vi "Periodic Tasks.vi"(8 "error in":errorcluster) -> ()   [LabVIEW 2019]
doc: "This VI runs in parallel to other tasks. It can contain as many user-defined periodic loops as you need. These can carry out PID or other sorts of timed response."
uses:
  Robot Global Data.vi
  <vilib>/Rock Robotics/Network Tables/NT Write Number.vi
  <vilib>/Rock Robotics/Network Tables/NT Read Number.vi
  <vilib>/Rock Robotics/Network Tables/NT Write Boolean.vi
  <vilib>/Rock Robotics/WPI/RobotDrive/WPI_RobotDriveArcadeDrive_Standard(NoSaturation).vi
  <vilib>/Rock Robotics/WPI/DriverStation/WPI_DriverStationRobotMode2.ctl
  <vilib>/Rock Robotics/Network Tables/NT Read Boolean.vi
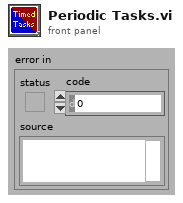
[diagram p1: front panel]
types:
  T1 = typedef "WPI_JoystickDevRef.ctl" = cluster{"Device":T2}
  T2 = typedef "WPI_JoystickDeviceEnum.ctl" = enum16{"USB 0", "USB 1", "USB 2", "USB 3", "USB 4", "USB 5"}
  T3 = typedef "WPI_RobotDriveDevRef.ctl" = cluster{"DevStatus":errorcluster, "Motors[]":T4[], "Square Inputs":bool, "Max Output":dbl}
  T4 = typedef "WPI_MotorControlDeviceRef.ctl" = cluster{"DeviceStatus":errorcluster, "Type":T5, "PWM":cluster{"PWM Channel":T6, "DeadBand":T7}, "CAN":cluster{"Device Number":u8, "SetOutput VI Ref":variant, "GetOutput VI Ref":variant, "Enable VI Ref":variant, "Disable VI Ref":variant, "Data":variant}, "Invert":bool, "DIO PWM":cluster{"PWM \"Enable\" Channel":T6, "DIOChannel":T8, "PWM Rate":dbl}}
  T5 = typedef "WPI_MotorControlType.ctl" = enum16{"PWM", "CAN", "DIO PWM"}
  T6 = typedef "FPGA_DIOPWMChannel.ctl" = enum8{"PWM 0", "PWM 1", "PWM 2", "PWM 3", "PWM 4", "PWM 5", "PWM 6", "PWM 7", "PWM 8", "PWM 9", "PWM MXP 0", "PWM MXP 1", "PWM MXP 2", "PWM MXP 3", "PWM MXP 4", "PWM MXP 5", "PWM MXP 6", "PWM MXP 7", "PWM MXP 8", "PWM MXP 9", "Invalid"}
  T7 = typedef "WPI_PWMDeadband.ctl" = cluster{"Name":string, "maxPositivePwm":i32, "minPositivePwm":i32, "centerPwm":i32, "maxNegativePwm":i32, "minNegativePwm":i32, "angularRange":u16}
  T8 = typedef "FPGA_DIOChannel.ctl" = enum8{"DIO 0", "DIO 1", "DIO 2", "DIO 3", "DIO 4", "DIO 5", "DIO 6", "DIO 7", "DIO 8", "DIO 9", "DIO MXP 0", "DIO MXP 1", "DIO MXP 2", "DIO MXP 3", "DIO MXP 4", "DIO MXP 5", "DIO MXP 6", "DIO MXP 7", "DIO MXP 8", "DIO MXP 9", "DIO MXP 10", "DIO MXP 11", "DIO MXP 12", "DIO MXP 13", "DIO MXP 14", "DIO MXP 15", "SPI Port CS1", "SPI Port CS2", "SPI Port CS3", "SPI Port MISO", "SPI Port MOSI", "Invalid"}
  T9 = cluster{"JoystickDevRef":T1, "RobotDriveDevRef":T3}
  T10 = typedef "WPI_DriverStationRobotMode2.ctl" = enum16{"Autonomous Disabled", "Autonomous Enabled", "Teleop Disabled", "Teleop Enabled", "Disconnected", "Finish", "Test Disabled", "Test Enabled", "Emergency Stopped"}
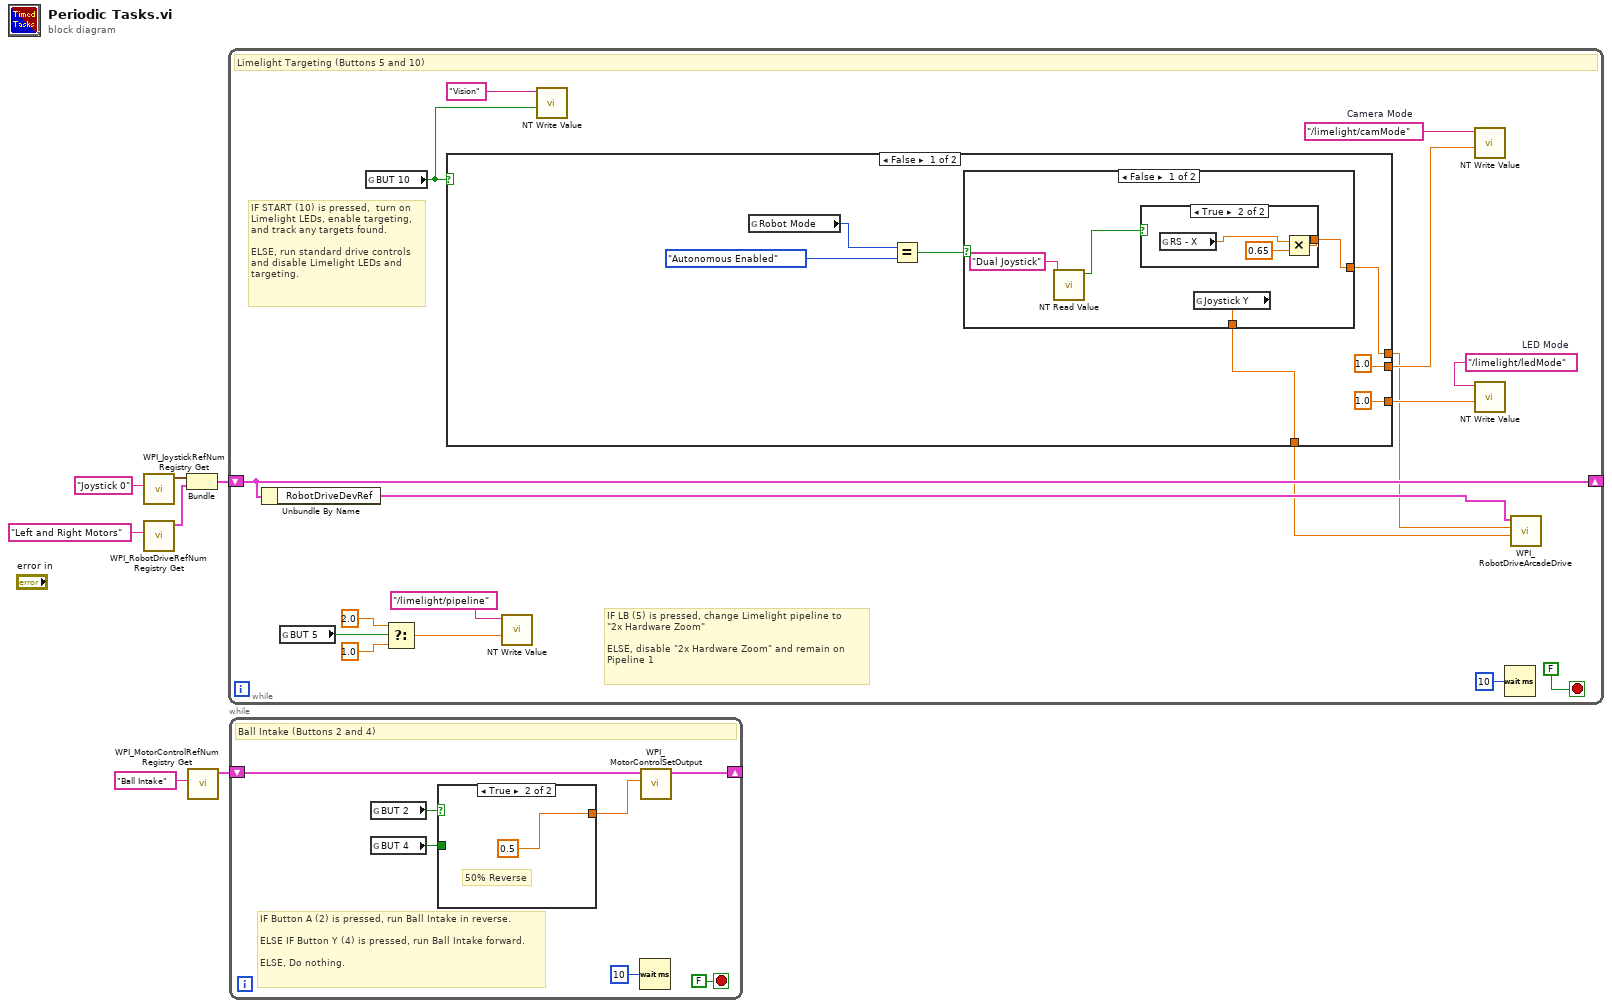
[diagram p0: block diagram]
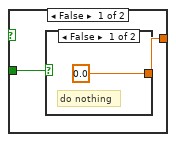
[diagram p2: hidden frame]
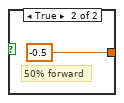
[diagram p3: hidden frame]
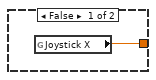
[diagram p4: hidden frame]
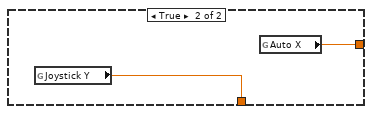
[diagram p5: hidden frame]
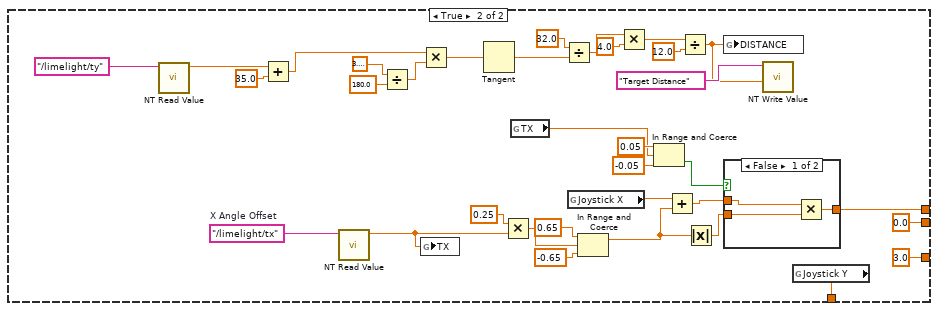
[diagram p6: hidden frame]
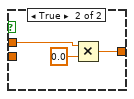
[diagram p7: hidden frame]
diagram:
  n1 = call <vilib>:"WPI_JoystickRefNum Registry Get.vi"("refnum name"="Joystick 0") -> ("JoystickDevRef"=w5:T1)  [unwired: 1 in, 9 out]
  n2 = call <vilib>:"WPI_RobotDriveRefNum Registry Get.vi"("refnum name"="Left and Right Motors") -> ("RobotDriveDevRef"=w4:T3)  [unwired: 1 in, 9 out]
  n3 = Bundle("JoystickDevRef"=w5, "RobotDriveDevRef"=w4) -> (w3:T9)  [unwired: 1 out]
  n4 = call <vilib>:"WPI_MotorControlRefNum Registry Get.vi"("refnum name"="Ball Intake") -> ("MotorControlDevRef"=w2:T4)  [unwired: 9 in, 1 out]
  n5 = while {
    shift-right: [w23] -> _
    shift-left: w3 -> [w23]
    stop <- FALSE stop-if-true
    w20 = "/limelight/camMode"  # Camera Mode
    w21 = "/limelight/ledMode"  # LED Mode
    # "IF LB (5) is pressed, change Limelight pipeline to \n\"2x Hardware Zoom\"\n\nELSE, disable \"2x Hardware Zoom\" and remain on\nPipeline 1"
    # "IF START (10) is pressed,  turn on\nLimelight LEDs, enable targeting,\nand track any targets found.\n\nELSE, run standard drive controls\nand disable Limelight LEDs and \ntargeting."
    # "Limelight Targeting (Buttons 5 and 10)"
    n6 = Unbundle By Name(w23) -> ("RobotDriveDevRef"=w22:T3)
    n7 = global read "Robot Global Data.vi" "BUT 5"() -> (w10:bool)
    n8 = global read "Robot Global Data.vi" "BUT 10"() -> (w16:bool)
    n9 = Select(t=2.0, s=w10, f=1.0) -> (s? t:f=w13:dbl)
    n10 = case shown="False" w16 {
      tunnel: [1.0 ("Numeric") 0.0 ("Numeric")] -> w19
      tunnel: [1.0 ("Numeric") 3.0 ("Numeric")] -> w18
      tunnel: [w25 w52] -> w8
      tunnel: [w29 w51] -> w9
      frame False {
        n11 = global read "Robot Global Data.vi" "Robot Mode"() -> (w28:T10)
        n12 = Equal?(x=w28, y=WPI_DriverStationRobotMode2."Autonomous Enabled") -> (x = y?=w26:bool)
        n13 = case shown="False" w26 {
          tunnel: [w33 w41] -> w29
          tunnel: [w32 w40] -> w25
          frame False {
            n14 = call-poly <vilib>:"NT Read Value.vi"("Name"="Dual Joystick") -> ("Boolean"=w34:bool)  [unwired: 9 in, 1 out]
            n15 = case shown="True" w34 {
              tunnel: [w36 w37] -> w32
              frame False {
                n16 = global read "Robot Global Data.vi" "Joystick X"() -> (w36:dbl)
              }
              frame True {
                n17 = global read "Robot Global Data.vi" "RS - X"() -> (w38:dbl)
                n18 = Multiply(x=w38, y=0.65) -> (x*y=w37:dbl)
              }
            }
            n19 = global read "Robot Global Data.vi" "Joystick Y"() -> (w33:dbl)
          }
          frame True {
            n20 = global read "Robot Global Data.vi" "Joystick Y"() -> (w41:dbl)
            n21 = global read "Robot Global Data.vi" "Auto X"() -> (w40:dbl)
          }
        }
      }
      frame True {
        w53 = "/limelight/tx"  # X Angle Offset
        n22 = call-poly <vilib>:"NT Read Value.vi"("Name"="/limelight/ty") -> ("Numeric"=w68:dbl)  [unwired: 9 in, 1 out]
        n23 = Add(x=w68, y=35.0) -> (x+y=w66:dbl)
        n24 = call-poly <vilib>:"NT Read Value.vi"("Name"=w53) -> ("Numeric"=w57:dbl)  [unwired: 9 in, 1 out]
        n25 = Divide(x=3.141592653589793, y=180.0) -> (x/y=w69:dbl)
        n26 = Multiply(x=w66, y=w69) -> (x*y=w65:dbl)
        n27 = global write "Robot Global Data.vi" "TX"(w57) -> ()
        n28 = Tangent(1:w65) -> (0:w75:dbl)
        n29 = Multiply(x=0.25 ("y"), y=w57) -> (x*y=w54:dbl)
        n30 = global read "Robot Global Data.vi" "TX"() -> (w47:dbl)
        n31 = Divide(x=32.0, y=w75) -> (x/y=w64:dbl)
        n32 = global read "Robot Global Data.vi" "Joystick X"() -> (w45:dbl)
        n33 = In Range and Coerce(upper limit=0.65, x=w54, lower limit=-0.65) -> (coerced(x)=w42:dbl)  [unwired: 1 out]
        n34 = Multiply(x=w64, y=4.0) -> (x*y=w62:dbl)
        n35 = In Range and Coerce(upper limit=0.05, x=w47, lower limit=-0.05) -> (In Range?=w50:bool)  [unwired: 1 out]
        n36 = Add(x=w45, y=w42) -> (x+y=w44:dbl)
        n37 = Divide(x=w62, y=12.0) -> (x/y=w58:dbl)
        n38 = Absolute Value(x=w42) -> (abs(x)=w43:dbl)
        n39 = global write "Robot Global Data.vi" "DISTANCE"(w58) -> ()
        n40 = case shown="False" w50 {
          tunnel: [w78 w80] -> w52
          tunnel: w44 -> [w77 w79]
          tunnel: w43 -> [w76 _]
          frame False {
            n41 = Multiply(x=w77, y=w76) -> (x*y=w78:dbl)
          }
          frame True {
            n42 = Multiply(x=w79, y=0.0) -> (x*y=w80:dbl)
          }
        }
        n43 = call-poly <vilib>:"NT Write Value.vi"("Numeric"=w58, "Name"="Target Distance") -> ()  [unwired: 9 in, 1 out]
        n44 = global read "Robot Global Data.vi" "Joystick Y"() -> (w51:dbl)
      }
    }
    n45 = call-poly <vilib>:"NT Write Value.vi"("Numeric"=w13, "Name"="/limelight/pipeline") -> ()  [unwired: 9 in, 1 out]
    n46 = call-poly <vilib>:"NT Write Value.vi"("Boolean"=w16, "Name"="Vision") -> ()  [unwired: 9 in, 1 out]
    n47 = call-poly <vilib>:"NT Write Value.vi"("Numeric"=w19, "Name"=w20) -> ()  [unwired: 9 in, 1 out]
    n48 = call-poly <vilib>:"NT Write Value.vi"("Numeric"=w18, "Name"=w21) -> ()  [unwired: 9 in, 1 out]
    n49 = Wait (ms)(milliseconds to wait=u32 10) -> ()  [unwired: 1 out]
    n50 = call-poly <vilib>:"WPI_RobotDriveArcadeDrive.vi"("Y axis value"=w9, "X axis value"=w8, "RobotDriveDevRef"=w22) -> ()  [unwired: 6 in, 3 out]
  }
  n51 = while {
    shift-right: [w85] -> _
    shift-left: w2 -> [w84]
    stop <- FALSE stop-if-true
    # "IF Button A (2) is pressed, run Ball Intake in reverse. \n\nELSE IF Button Y (4) is pressed, run Ball Intake forward.\n\nELSE, Do nothing."
    # "Ball Intake (Buttons 2 and 4)"
    n52 = global read "Robot Global Data.vi" "BUT 2"() -> (w87:bool)
    n53 = global read "Robot Global Data.vi" "BUT 4"() -> (w88:bool)
    n54 = case shown="True" w87 {
      tunnel: [w90 0.5 ("Output")] -> w86
      tunnel: w88 -> [w89 _]
      frame False {
        n55 = case shown="False" w89 {
          tunnel: [0.0 ("Output") -0.5 ("Output")] -> w90
          frame False {
            # "do nothing"
          }
          frame True {
            # "50% forward"
          }
        }
      }
      frame True {
        # "50% Reverse"
      }
    }
    n56 = Wait (ms)(milliseconds to wait=u32 10) -> ()  [unwired: 1 out]
    n57 = call <vilib>:"WPI_MotorControlSetOutput.vi"("Output"=w86, "MotorControlDevRef"=w84) -> ("MotorControlDevRef"=w85:T4)  [unwired: 7 in, 2 out]
  }
